vi "Add MakerHub Feed.vi"(8 "Error In":errorcluster, 11 "Install LV Data":T1={"SSH Session"=refnum, "Status Log"="", "Detailed Log"="", "Credentials"={"Hostname or IP"="192.168.7.2", "Username"="root", "Password"=""}, "Target Info"={"OS Version"="", "CPU"="", "Systemd Version"="", "Internet Access"=FALSE, "Device Type"="", "LV Installed Ver"="", "LV Available Ver"="", "LV Upgrade Available"=FALSE, "Hostname"="", "NIC Info"=[]}, "Reboot Required?"=FALSE}) -> (0 "Error Out":errorcluster, 1 "Log":string, 3 "Install LV Data":T1={"SSH Session"=refnum, "Status Log"="", "Detailed Log"="", "Credentials"={"Hostname or IP"="192.168.7.2", "Username"="root", "Password"=""}, "Target Info"={"OS Version"="", "CPU"="", "Systemd Version"="", "Internet Access"=FALSE, "Device Type"="", "LV Installed Ver"="", "LV Available Ver"="", "LV Upgrade Available"=FALSE, "Hostname"="", "NIC Info"=[]}, "Reboot Required?"=FALSE})   [LabVIEW 2014, in "LMH-LINX.lvlib"]
uses:
  <vilib>/MakerHub/LINX/LMH-LINX.lvlib
  <vilib>/MakerHub/LINX/Private/Utilties/Target Management/Install LV Data.ctl
  C:/Program Files (x86)/National Instruments/LabVIEW 2014/vi.lib/MakerHub/LINX/Resources/Renci.SshNet.dll
  Resources/Renci.SshNet.dll
  <vilib>/MakerHub/LINX/Private/Utilties/Target Management/Target Info.ctl
  <vilib>/MakerHub/LINX/Private/Utilties/Target Management/NIC Info.ctl
  <vilib>/MakerHub/LINX/Private/Utilties/Target Management/NIC Mode.ctl
  <vilib>/regexp/Match Regular Expression.xnode
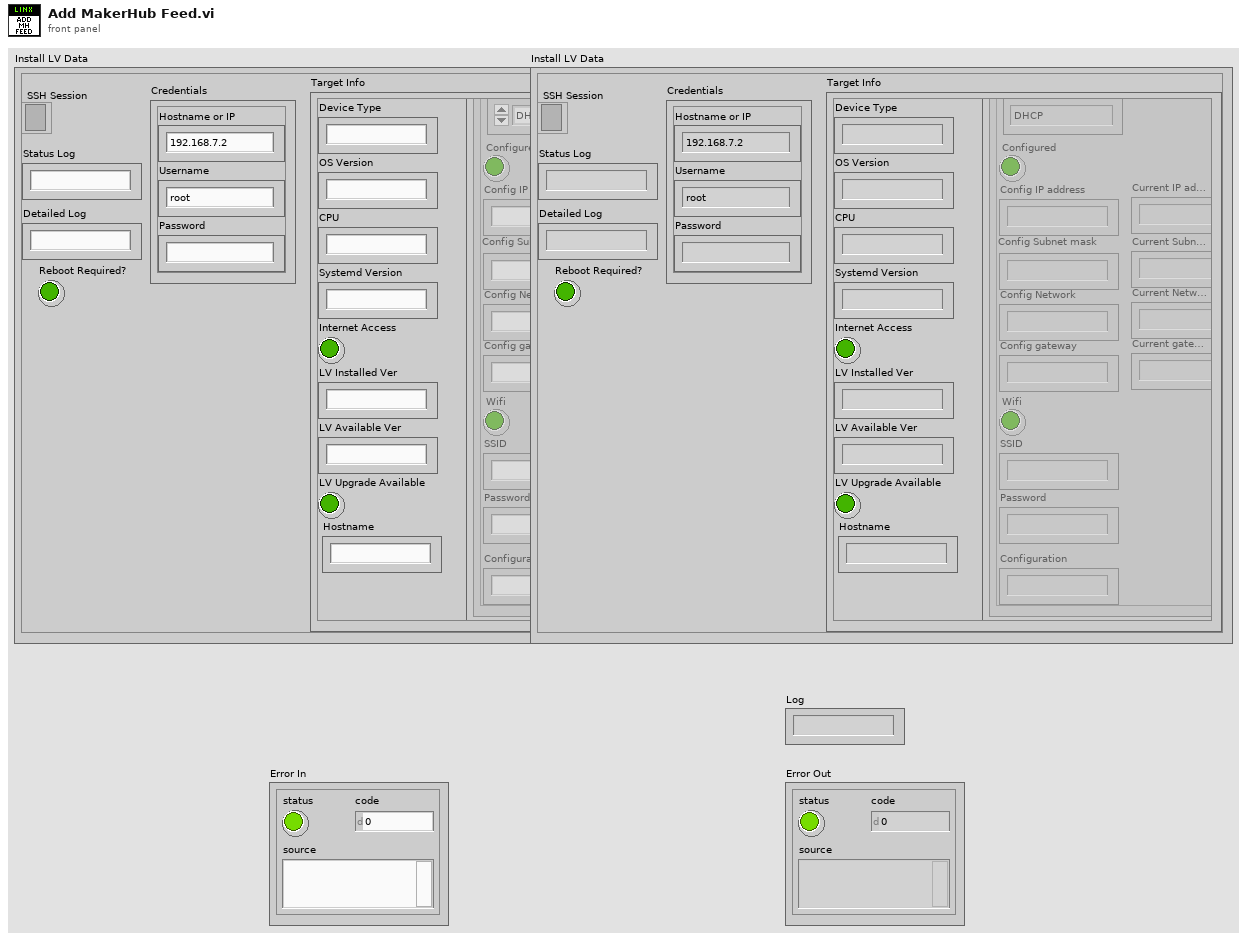
[diagram p1: front panel]
types:
  T1 = typedef "LMH-LINX.lvlib/Install LV Data.ctl" = cluster{"SSH Session":refnum<k24>, "Status Log":string, "Detailed Log":string, "Credentials":cluster{"Hostname or IP":string, "Username":string, "Password":string}, "Target Info":T2, "Reboot Required?":bool}
  T2 = typedef "LMH-LINX.lvlib/Target Info.ctl" = cluster{"OS Version":string, "CPU":string, "Systemd Version":string, "Internet Access":bool, "Device Type":string, "LV Installed Ver":string, "LV Available Ver":string, "LV Upgrade Available":bool, "Hostname":string, "NIC Info":T3[]}
  T3 = typedef "LMH-LINX.lvlib/NIC Info.ctl" = cluster{"Name":string, "NIC Mode":T4, "Configured":bool, "Config IP address":string, "Config Subnet mask":string, "Config Network":string, "Config gateway":string, "Wifi":bool, "SSID":string, "Password":string, "Configuration":string, "Current IP address":string, "Current Subnet mask":string, "Current gateway":string, "Current Network":string}
  T4 = typedef "LMH-LINX.lvlib/NIC Mode.ctl" = enum16{"DHCP", "Static", "Loopback"}
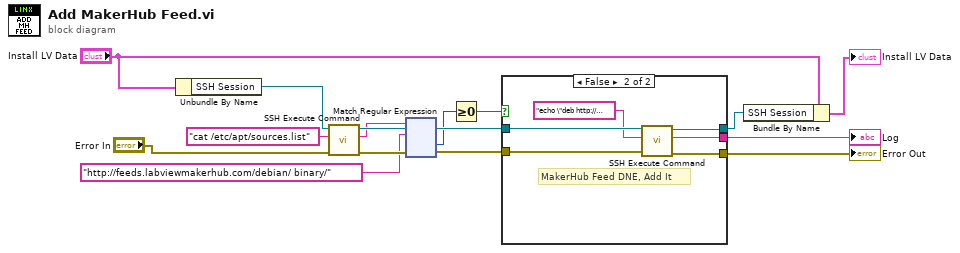
[diagram p0: block diagram]
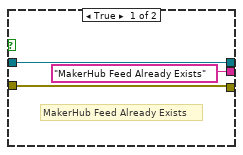
[diagram p2: hidden frame]
diagram:
  n1 = Unbundle By Name("Install LV Data") -> ("SSH Session"=w10:refnum<k24>)
  n2 = call <vilib>:"SSH Execute Command.vi"("Error In"="Error In", "Command"="cat /etc/apt/sources.list", "SSH Session"=w10) -> ("Error Out"=w5:errorcluster, "Std Out"=w6:string, "SSH Session"=w7:refnum<k24>)  [unwired: 6 in]
  n3 = xnode "Match Regular Expression"("input string"=w6, "regular expression"="http://feeds.labviewmakerhub.com/debian/ binary/", "error in"=w5) -> ("offset past match"=w2:i32, "error out"=w4:errorcluster)  [unwired: 3 in, 3 out]
  n4 = Greater Or Equal To 0?(x=w2) -> (x >= 0?=w1:bool)
  n5 = case shown="False" w1 {
    tunnel: ["MakerHub Feed Already Exists" ("Std Out") w24] -> w15
    tunnel: [w18 w23] -> w14
    tunnel: [w16 w22] -> w13
    tunnel: w7 -> [w16 w21]
    tunnel: w4 -> [w18 w20]
    frame True {
      # "MakerHub Feed Already Exists"
    }
    frame False {
      # "MakerHub Feed DNE, Add It"
      n6 = call <vilib>:"SSH Execute Command.vi"("Error In"=w20, "Command"="echo \"deb http://feeds.labviewmakerhub.com/debian/ binary/\" | sudo tee -a /etc/apt/sources.list", "SSH Session"=w21) -> ("Error Out"=w23:errorcluster, "Std Out"=w24:string, "SSH Session"=w22:refnum<k24>)  [unwired: 6 in]
    }
  }
  "Log" <- w15
  "Error Out" <- w14
  n7 = Bundle By Name(cluster="Install LV Data", "SSH Session"=w13) -> (→"Install LV Data":T1)
